vi "cmd_delay.vi"(8 "error in (no error)":errorcluster, 10 "command delay (ms)":u32=100, 11 "VISA Refnum in":refnum<visa-resource-name>) -> (0 "error out":errorcluster, 3 "VISA Refnum out":refnum<visa-resource-name>)   [LabVIEW 2018]
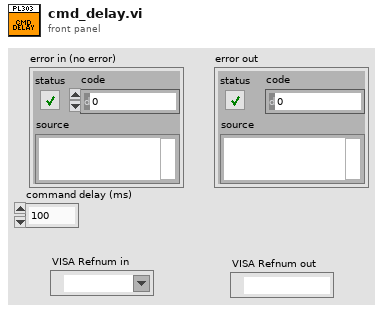
[diagram p1: front panel]
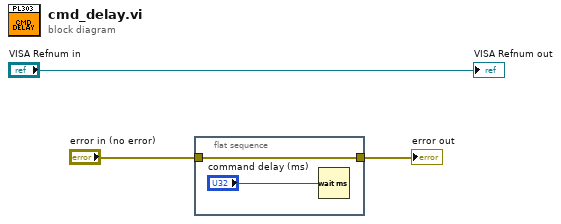
[diagram p0: block diagram]
diagram:
  n1 = flat-sequence {
    tunnel: [w4] -> w2
    tunnel: "error in (no error)" -> [w4]
    frame #0 {
      n2 = Wait (ms)(milliseconds to wait="command delay (ms)") -> ()  [unwired: 1 out]
    }
  }
  "error out" <- w2
  "VISA Refnum out" <- "VISA Refnum in"
